vi "Open Config Data.vi"(8 "error in (no error)":errorcluster, 10 "create file if necessary (T)":bool=TRUE, 11 "configuration file path":path) -> (0 "error out":errorcluster, 2 "file created?":bool, 3 "refnum":T1)   [LabVIEW 2010, in "NI_LVConfig.lvlib"]
doc: "Opens a reference to the configuration data found in a platform-independent configuration file."
uses:
  NI_LVConfig.lvlib
  Config Data RefNum.ctl
  Config Data.ctl
  Section.ctl
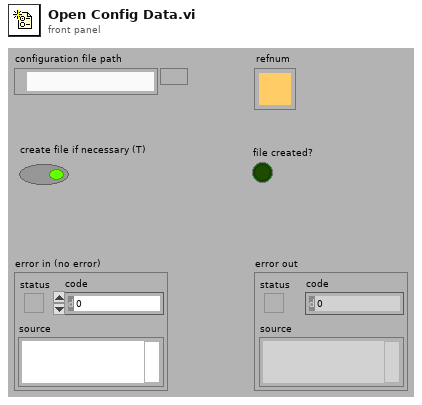
[diagram p1: front panel]
types:
  T1 = typedef "NI_LVConfig.lvlib/Config Data RefNum.ctl" = refnum<k1>
  T2 = typedef "NI_LVConfig.lvlib/Config Data.ctl" = cluster{"sections":T3[], "path":path, "dirty":bool}
  T3 = typedef "NI_LVConfig.lvlib/Section.ctl" = cluster{"name":string, "comment":string, "kvc":string[][]}
  T4 = typedef "NI_LVConfig.lvlib/Config Queue.ctl" = refnum<queue>
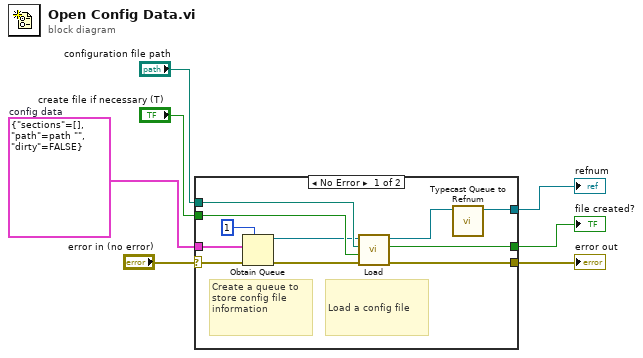
[diagram p0: block diagram]
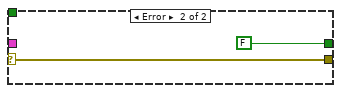
[diagram p2: hidden frame]
diagram:
  w1 = T2 {"sections"=[], "path"=path "", "dirty"=FALSE}  # config data
  n1 = case shown="No Error" "error in (no error)" {
    selector: "error in (no error)" -> [w13 w20]
    tunnel: "configuration file path" -> [w18 _]
    tunnel: "create file if necessary (T)" -> [w17 _]
    tunnel: [w15 FALSE ("file created?")] -> w3
    tunnel: [w16 w20] -> w4
    tunnel: w1 -> [w12 _]
    tunnel: [w9 _] -> w2
    frame No Error {
      # "Load a config file"
      # "Create a queue to store config file information"
      n2 = Obtain Queue(max queue size (-1, unlimited)=1, element data type=w12, error in (no error)=w13) -> (queue out=w8:refnum<queue>, error out=w11:errorcluster)  [unwired: 2 in, 1 out]
      n3 = call "Load.vi"("error in (no error)"=w11, "create file if necessary? (T)"=w17, "configuration file path"=w18, "queue in"=w8) -> ("error out"=w16:errorcluster, "file created?"=w15:bool, "queue out"=w10:T4)  [unwired: 1 in, 4 out]
      n4 = call "Typecast Queue to Refnum.vi"("queue in"=w10) -> ("refnum out"=w9:T1)  [unwired: 10 in]
    }
    frame Error {
    }
  }
  "error out" <- w4
  "file created?" <- w3
  "refnum" <- w2
